vi "Periodic Tasks.vi"(8 "error in":errorcluster) -> ()   [LabVIEW 2014]
doc: "This VI runs in parallel to other tasks. It can contain as many user-defined periodic loops as you need. These can carry out PID or other sorts of timed response."
uses:
  <vilib>/Rock Robotics/WPI/Joystick/WPI_JoystickGetSetRefNum.vi
  <vilib>/Rock Robotics/WPI/RobotDrive/WPI_RobotDriveGetSetRefNum.vi
panel:
  out "Right Continuer":bool
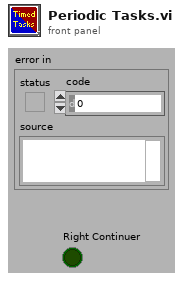
[diagram p1: front panel]
types:
  T1 = typedef "WPI_JoystickDevRef.ctl" = cluster{"Device":T2}
  T2 = typedef "WPI_JoystickDeviceEnum.ctl" = enum16{"USB 0", "USB 1", "USB 2", "USB 3", "USB 4", "USB 5"}
  T3 = typedef "WPI_RobotDriveDevRef.ctl" = cluster{"DevStatus":errorcluster, "Motors[]":T4[], "Square Inputs":bool, "Max Output":dbl}
  T4 = typedef "WPI_MotorControlDeviceRef.ctl" = cluster{"DeviceStatus":errorcluster, "Type":T5, "PWM":cluster{"Controller":T6, "PWM Channel":T7, "DeadBand":T8}, "CAN":cluster{"Device Number":u8, "Control Mode":T9, "Semaphore":T10, "Max Vout":dbl, "TalonSRX Control Mode":T11}, "Invert":bool, "TransformRef":T12, "InvTransformRef":T12}
  T5 = typedef "WPI_MotorControlType.ctl" = enum16{"PWM", "CAN", "CANTalonSRX"}
  T6 = typedef "FPGA_TypedefDigitalModule.ctl" = enum16{"Controller 1"}
  T7 = typedef "FPGA_DIOPWMChannel.ctl" = enum8{"PWM 0", "PWM 1", "PWM 2", "PWM 3", "PWM 4", "PWM 5", "PWM 6", "PWM 7", "PWM 8", "PWM 9", "PWM MXP 0", "PWM MXP 1", "PWM MXP 2", "PWM MXP 3", "PWM MXP 4", "PWM MXP 5", "PWM MXP 6", "PWM MXP 7", "PWM MXP 8", "PWM MXP 9", "Invalid"}
  T8 = typedef "WPI_PWMDeadband.ctl" = cluster{"Name":string, "maxPositivePwm":i32, "minPositivePwm":i32, "centerPwm":i32, "maxNegativePwm":i32, "minNegativePwm":i32, "angularRange":u16}
  T9 = typedef "WPI_CANJaguar_ControlMode.ctl" = enum8{"Percent VBus", "Current", "Speed", "Position", "Voltage"}
  T10 = typedef "Semaphore RefNum" = refnum<k1>
  T11 = typedef "WPI_CANTalonSRX_APIControlMode.ctl" = enum8{"Percent VBus", "Speed", "Position", "Slave", "Unchanged / Invalid"}
  T12 = typedef "WPI_PWMTransform_ConPane.ctl" = refnum<vi>
  T13 = cluster{"JoystickDevRef":T1, "JoystickDevRef":T1, "RobotDriveDevRef":T3}
  T14 = cluster{"Buttons[0]":bool, "Buttons[1]":bool, "Buttons[2]":bool, "Buttons[3]":bool, "Buttons[4]":bool, "Buttons[5]":bool, "Buttons[6]":bool, "Buttons[7]":bool, "Buttons[8]":bool}
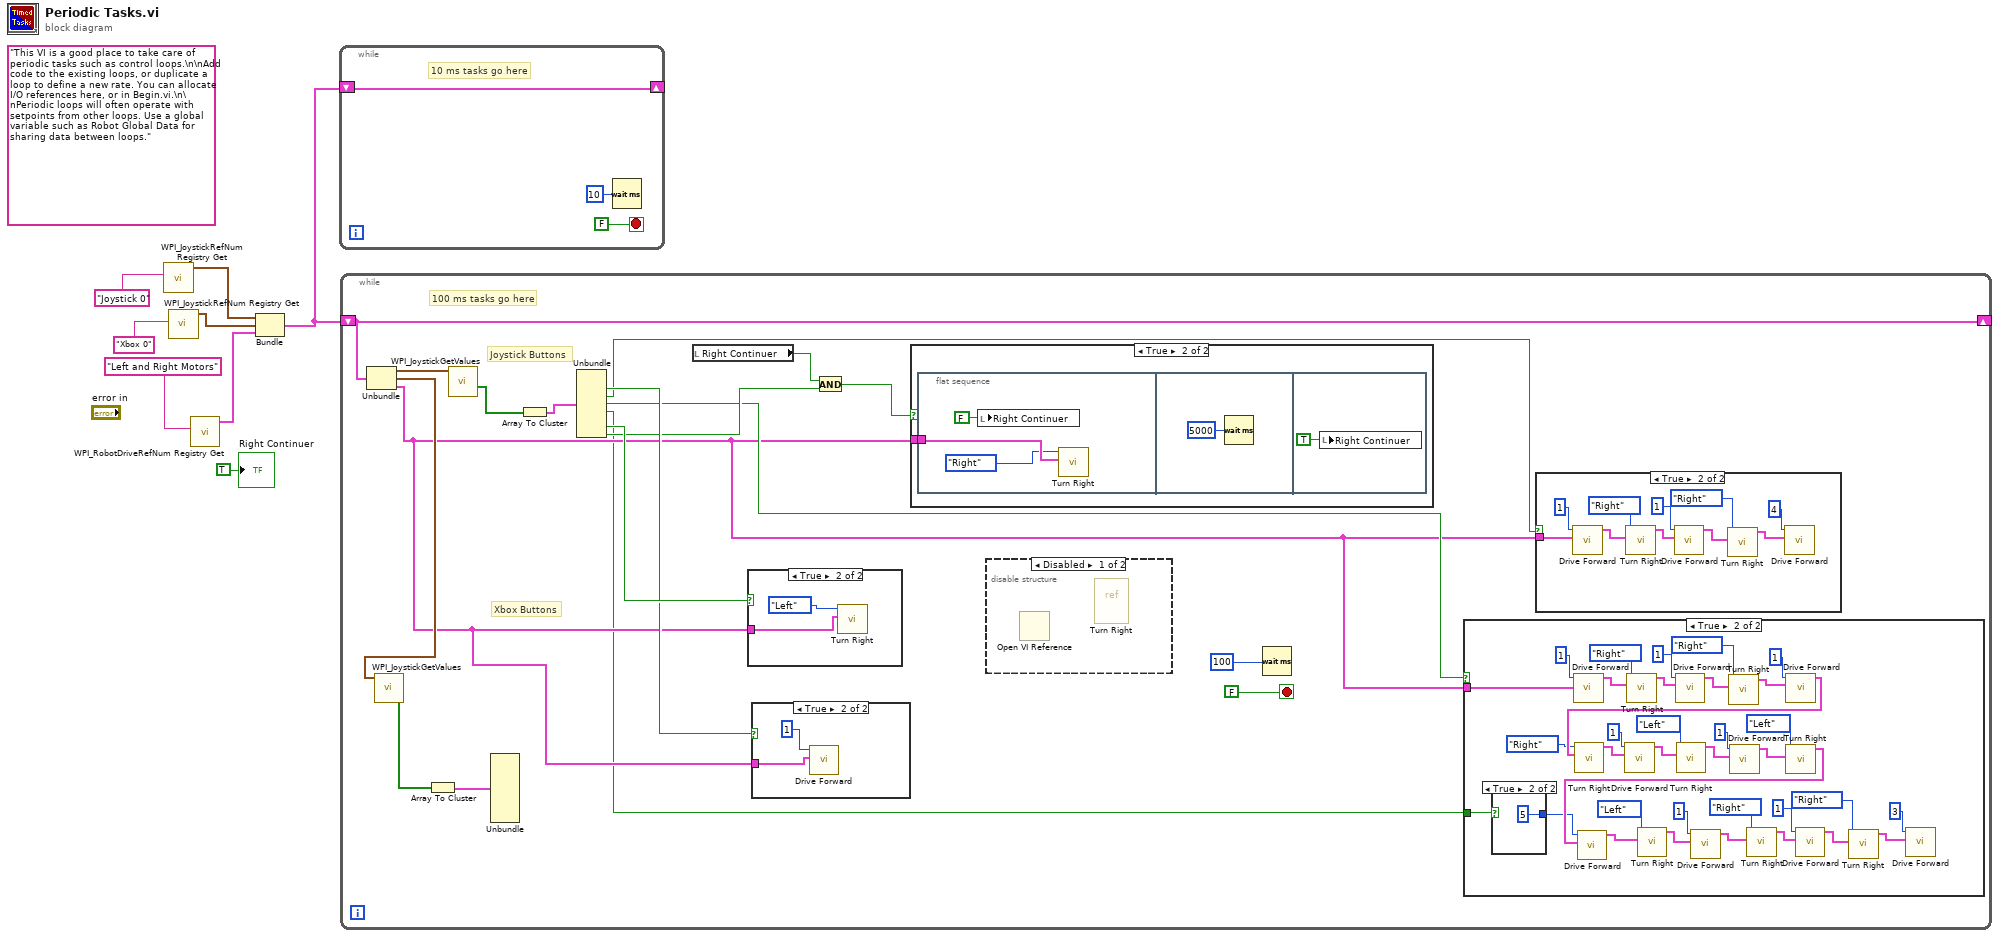
[diagram p0: block diagram]
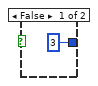
[diagram p4: hidden frame]
diagram:
  (unwired) "This VI is a good place to take care of periodic tasks such as control loops.\n\nAdd code to the existing loops, or duplicate a loop to define a new rate. You can allocate I/O references here, or in Begin.vi.\n\nPeriodic loops will often operate with setpoints from other loops. Use a global variable such as Robot Global Data for sharing data between loops."
  n1 = call <vilib>:"WPI_JoystickRefNum Registry Get.vi"("refnum name"="Joystick 0") -> ("JoystickDevRef"=w6:T1)  [unwired: 1 in, 9 out]
  n2 = call <vilib>:"WPI_JoystickRefNum Registry Get.vi"("refnum name"="Xbox 0") -> ("JoystickDevRef"=w2:T1)  [unwired: 1 in, 9 out]
  n3 = call <vilib>:"WPI_RobotDriveRefNum Registry Get.vi"("refnum name"="Left and Right Motors") -> ("RobotDriveDevRef"=w4:T3)  [unwired: 1 in, 9 out]
  n4 = Bundle("JoystickDevRef"=w6, "JoystickDevRef"=w2, "RobotDriveDevRef"=w4) -> (w5:T13)  [unwired: 1 out]
  n5 = while {
    shift-right: [w9] -> _
    shift-left: w5 -> [w9]
    stop <- FALSE stop-if-true
    # "10 ms tasks go here"
    n6 = Wait (ms)(milliseconds to wait=u32 10) -> ()  [unwired: 1 out]
  }
  n7 = while {
    shift-right: [w28] -> _
    shift-left: w5 -> [w28]
    stop <- FALSE stop-if-true
    # "Joystick Buttons"
    # "Xbox Buttons"
    # "100 ms tasks go here"
    n8 = Unbundle(w28) -> ("JoystickDevRef"=w27:T1, "JoystickDevRef"=w26:T1, "RobotDriveDevRef"=w14:T3)
    n9 = call <vilib>:"WPI_JoystickGetValues.vi"("JoystickDevRef"=w26) -> ("Buttons"=w23:bool[])  [unwired: 6 in, 4 out]
    n10 = Array To Cluster(array=w23) -> (cluster=w22:T14)
    n11 = call <vilib>:"WPI_JoystickGetValues.vi"("JoystickDevRef"=w27) -> ("Buttons"=w25:bool[])  [unwired: 6 in, 4 out]
    n12 = Unbundle(w22) -> ()  [unwired: 9 out]
    n13 = Array To Cluster(array=w25) -> (cluster=w24:T14)
    n14 = Unbundle(w24) -> ("Buttons[2]"=w20:bool, "Buttons[3]"=w12:bool, "Buttons[4]"=w15:bool, "Buttons[5]"=w13:bool, "Buttons[7]"=w21:bool, "Buttons[8]"=w19:bool)  [unwired: 3 out]
    n15 = local read "Right Continuer"() -> (w16:bool)
    n16 = case shown="True" w21 {
      tunnel: w14 -> [_ w79]
      frame False {
      }
      frame True {
        n17 = call "Turn Right.vi"("RobotDriveDevRef in"=w79, "Turn Direction"=enum16{"Right", "Left"}."Left") -> ()  [unwired: 9 in, 1 out]
      }
    }
    n18 = case shown="True" w20 {
      tunnel: w14 -> [_ w77]
      frame False {
      }
      frame True {
        n19 = call "Drive Forward.vi"("RobotDriveDevRef in"=w77, "Numeric"=1) -> ()  [unwired: 9 in, 1 out]
      }
    }
    n20 = And(x=w16, y=w19) -> (x .and. y?=w18:bool)
    n21 = case shown="True" w18 {
      tunnel: w14 -> [_ w81]
      frame False {
      }
      frame True {
        n22 = flat-sequence {
          tunnel: w81 -> [w84]
          frame #0 {
            n23 = local write "Right Continuer"(FALSE ("Right Continuer")) -> ()
            n24 = call "Turn Right.vi"("RobotDriveDevRef in"=w84, "Turn Direction"=enum16{"Right", "Left"}."Right") -> ()  [unwired: 9 in, 1 out]
          }
          frame #1 {
            n25 = Wait (ms)(milliseconds to wait=u32 5000) -> ()  [unwired: 1 out]
          }
          frame #2 {
            n26 = local write "Right Continuer"(TRUE ("Right Continuer")) -> ()
          }
        }
      }
    }
    n27 = disable-structure shown="Disabled" {
      frame Disabled {
        n28 = Open VI Reference() -> ()  [unwired: 6 in, 2 out]
        n29 = vi-ref "Turn Right.vi"() -> ()  [unwired: 1 out]
      }
      frame Enabled {
      }
    }
    n30 = Wait (ms)(milliseconds to wait=u32 100) -> ()  [unwired: 1 out]
    n31 = case shown="True" w15 {
      tunnel: w14 -> [_ w31]
      tunnel: w13 -> [_ w30]
      frame False {
      }
      frame True {
        n32 = case shown="True" w30 {
          tunnel: [3 ("Numeric") 5 ("Numeric")] -> w33
          frame False {
          }
          frame True {
          }
        }
        n33 = call "Drive Forward.vi"("RobotDriveDevRef in"=w31, "Numeric"=1) -> ("RobotDriveDevRef out"=w64:T3)  [unwired: 9 in]
        n34 = call "Turn Right.vi"("RobotDriveDevRef in"=w64, "Turn Direction"=enum16{"Right", "Left"}."Right") -> ("RobotDriveDevRef out"=w63:T3)  [unwired: 9 in]
        n35 = call "Drive Forward.vi"("RobotDriveDevRef in"=w63, "Numeric"=1) -> ("RobotDriveDevRef out"=w62:T3)  [unwired: 9 in]
        n36 = call "Turn Right.vi"("RobotDriveDevRef in"=w62, "Turn Direction"=enum16{"Right", "Left"}."Right") -> ("RobotDriveDevRef out"=w61:T3)  [unwired: 9 in]
        n37 = call "Drive Forward.vi"("RobotDriveDevRef in"=w61, "Numeric"=1) -> ("RobotDriveDevRef out"=w56:T3)  [unwired: 9 in]
        n38 = call "Turn Right.vi"("RobotDriveDevRef in"=w56, "Turn Direction"=enum16{"Right", "Left"}."Right") -> ("RobotDriveDevRef out"=w55:T3)  [unwired: 9 in]
        n39 = call "Drive Forward.vi"("RobotDriveDevRef in"=w55, "Numeric"=1) -> ("RobotDriveDevRef out"=w54:T3)  [unwired: 9 in]
        n40 = call "Turn Right.vi"("RobotDriveDevRef in"=w54, "Turn Direction"=enum16{"Right", "Left"}."Left") -> ("RobotDriveDevRef out"=w53:T3)  [unwired: 9 in]
        n41 = call "Drive Forward.vi"("RobotDriveDevRef in"=w53, "Numeric"=1) -> ("RobotDriveDevRef out"=w52:T3)  [unwired: 9 in]
        n42 = call "Turn Right.vi"("RobotDriveDevRef in"=w52, "Turn Direction"=enum16{"Right", "Left"}."Left") -> ("RobotDriveDevRef out"=w51:T3)  [unwired: 9 in]
        n43 = call "Drive Forward.vi"("RobotDriveDevRef in"=w51, "Numeric"=w33) -> ("RobotDriveDevRef out"=w45:T3)  [unwired: 9 in]
        n44 = call "Turn Right.vi"("RobotDriveDevRef in"=w45, "Turn Direction"=enum16{"Right", "Left"}."Left") -> ("RobotDriveDevRef out"=w47:T3)  [unwired: 9 in]
        n45 = call "Drive Forward.vi"("RobotDriveDevRef in"=w47, "Numeric"=1) -> ("RobotDriveDevRef out"=w34:T3)  [unwired: 9 in]
        n46 = call "Turn Right.vi"("RobotDriveDevRef in"=w34, "Turn Direction"=enum16{"Right", "Left"}."Right") -> ("RobotDriveDevRef out"=w41:T3)  [unwired: 9 in]
        n47 = call "Drive Forward.vi"("RobotDriveDevRef in"=w41, "Numeric"=1) -> ("RobotDriveDevRef out"=w40:T3)  [unwired: 9 in]
        n48 = call "Turn Right.vi"("RobotDriveDevRef in"=w40, "Turn Direction"=enum16{"Right", "Left"}."Right") -> ("RobotDriveDevRef out"=w39:T3)  [unwired: 9 in]
        n49 = call "Drive Forward.vi"("RobotDriveDevRef in"=w39, "Numeric"=3) -> ()  [unwired: 9 in, 1 out]
      }
    }
    n50 = case shown="True" w12 {
      tunnel: w14 -> [_ w67]
      frame False {
      }
      frame True {
        n51 = call "Drive Forward.vi"("RobotDriveDevRef in"=w67, "Numeric"=1) -> ("RobotDriveDevRef out"=w76:T3)  [unwired: 9 in]
        n52 = call "Turn Right.vi"("RobotDriveDevRef in"=w76, "Turn Direction"=enum16{"Right", "Left"}."Right") -> ("RobotDriveDevRef out"=w75:T3)  [unwired: 9 in]
        n53 = call "Drive Forward.vi"("RobotDriveDevRef in"=w75, "Numeric"=1) -> ("RobotDriveDevRef out"=w74:T3)  [unwired: 9 in]
        n54 = call "Turn Right.vi"("RobotDriveDevRef in"=w74, "Turn Direction"=enum16{"Right", "Left"}."Right") -> ("RobotDriveDevRef out"=w73:T3)  [unwired: 9 in]
        n55 = call "Drive Forward.vi"("RobotDriveDevRef in"=w73, "Numeric"=4) -> ()  [unwired: 9 in, 1 out]
      }
    }
  }
  "Right Continuer" <- TRUE ("Right Continuer")
